vi "Hysteresis.vi"() -> ()   [LabVIEW 2016]
uses:
  controls/HysteresisCtl.ctl
  controls/Enum.ctl
  libgwyscan-1.2-labview2015-win32/controls/parameters for save Gwyddion arrays.ctl
  <vilib>/Analysis/baseanly.llb/Mean (DBL).vi
  <vilib>/Utility/file.llb/Read Delimited Spreadsheet (string).vi
  <vilib>/Utility/error.llb/Error Cluster From Error Code.vi
  <vilib>/rvi/errors/niLvFpgaAdjustHostInterfaceError.vi
  <vilib>/rvi/interface/nirviReadWriteControl/nirviReadWriteControl.xnode
  controls/FPGAVIreferenceTypeDef.ctl
  FPGA Bitfiles/qnmController797_usbRIO_controllerFPGAmu.lvbitx
  <vilib>/Analysis/NI_AALBase.lvlib
  <vilib>/Analysis/NI_AALPro.lvlib
  NiFpgaLv.dll
panel:
  out "bwd":dbl[](array[numeric]) format="%#.4g"
  in  "Processing":u16(ring) items=["None", "Offset", "Line", "Polynom"]
  in  "Frame":bool=TRUE
  in  "rel Range":dbl=1.0 format="%#_13g"
  in  "fwd":path
  in  "bwd":path
  out "Corrected":T1
  out "Raw":cluster{"fwd raw":dbl[][], "bwd raw":dbl[][]}
  in  "Picture Parameters (to save)":T2={"Width"=0.000136, "Height"=0.000136, "Pixels/Line"=0.0, "Lines"=0.0}
  in  "Data source":enum32{"File", "Internal"}(radio)
  in  "Save":bool
  out "fwd":dbl[](array[numeric]) format="%#.4g"
  in  "Update Hysteresis":bool
  in  "Upload":bool
  in  "Hypothesis":T3(ring)=enum."2nd esti"
  in  "Display Correction":bool
  # "Polynom\ncoeff : a+bx\n+cx2+dx3"
  # "up"
  # "down"
  # "Path (txt/dat)"
  # "Corrected"
  # "Raw"
  # "Forward"
  # "Backward"
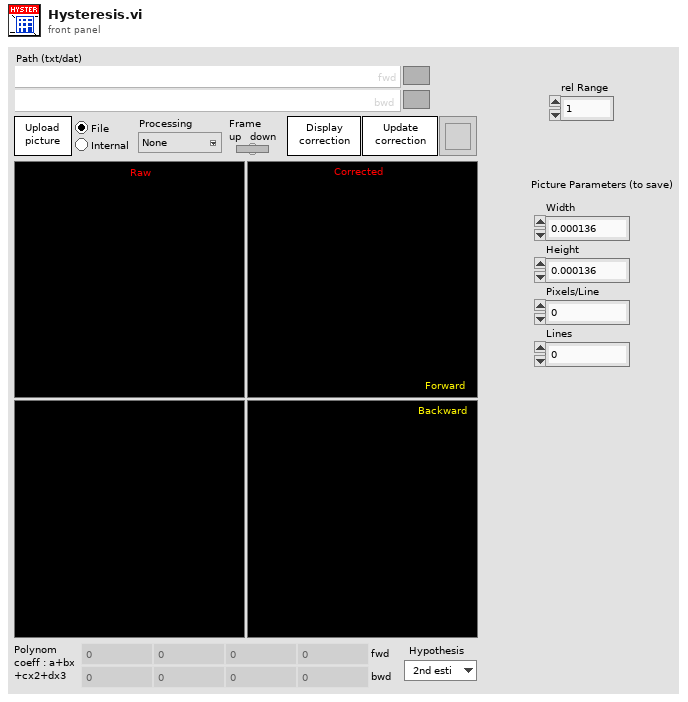
[diagram p1: front panel]
types:
  T1 = cluster{"fwd corrected":dbl[][], "bwd corrected":dbl[][]}
  T2 = cluster{"Width":dbl, "Height":dbl, "Pixels/Line":dbl, "Lines":dbl}
  T3 = enum16{"bwd", "middle", "fwd", "linear", "2nd esti"}
  T4 = typedef "HysteresisCtl.ctl" = enum16{"Init", "Display Correction", "Upload Picture", "Update Hysteresis", "WaitForEvents", "Change.Hypothesis", "Save", "Close"}
  T5 = typedef "Enum.ctl" = enum16{"Init", "Read", "Write"}
  T6 = cluster{"write":bool, "index":u16, "data":fxp<+/-,18,5>}
  T7 = typedef "parameters for save Gwyddion arrays.ctl" = cluster{"X res":i32, "Y res ":i32, "xreal":dbl, "yreal":dbl, "nChannels":i32, "filename":string, "Descriptions":string[], "xyunit":string[], "Z unit":string[]}
  T8 = cluster{"Waveform Shape Fast In":dbl[], "Waveform Shape Slow In":dbl[]}
  T9 = typedef "FPGAVIreferenceTypeDef.ctl" = refnum<k20>
  T10 = cluster{"se.p.enable":bool, "se.p.singleDirection":bool, "se.p.haltScan":bool, "se.mot.p.start":bool}
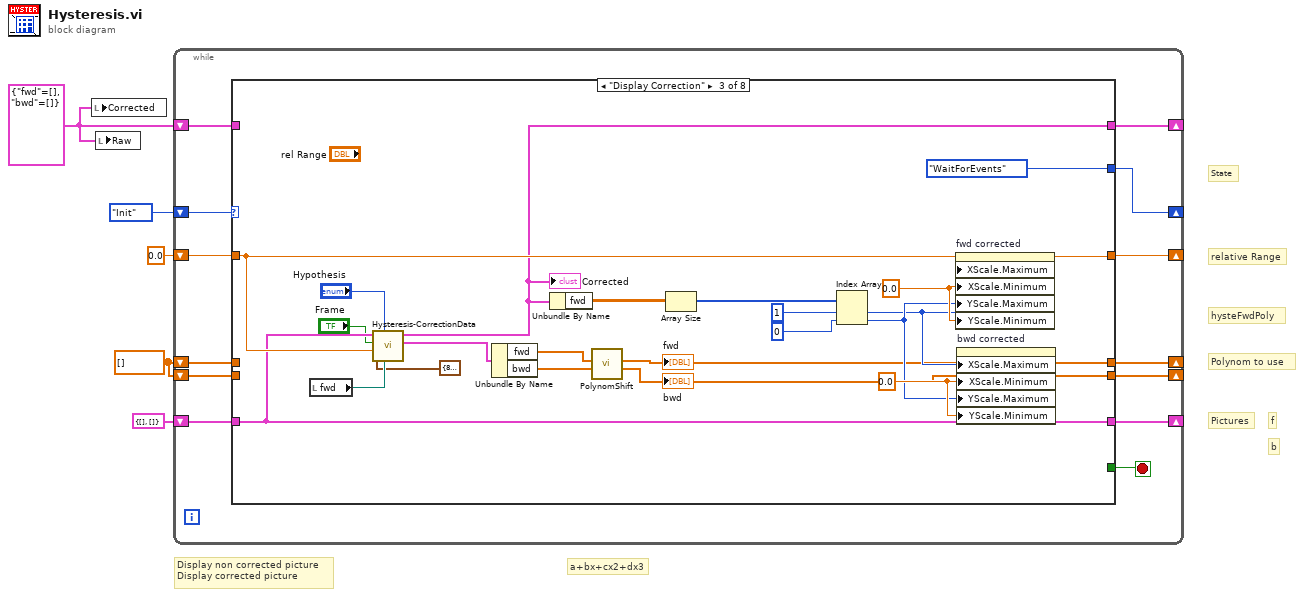
[diagram p0: block diagram]
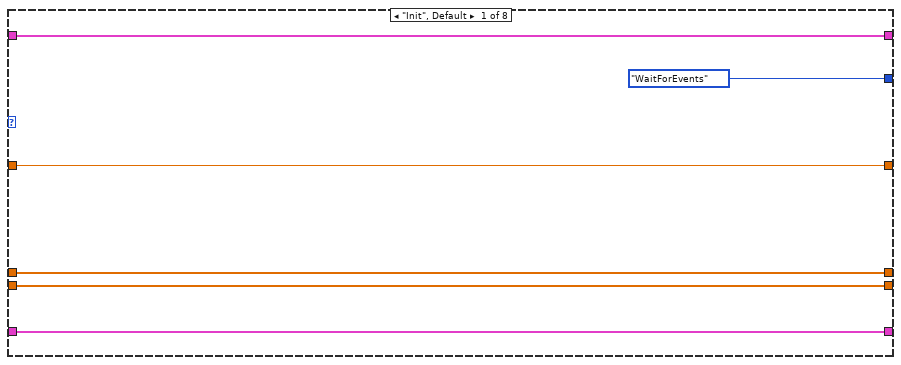
[diagram p2: hidden frame]
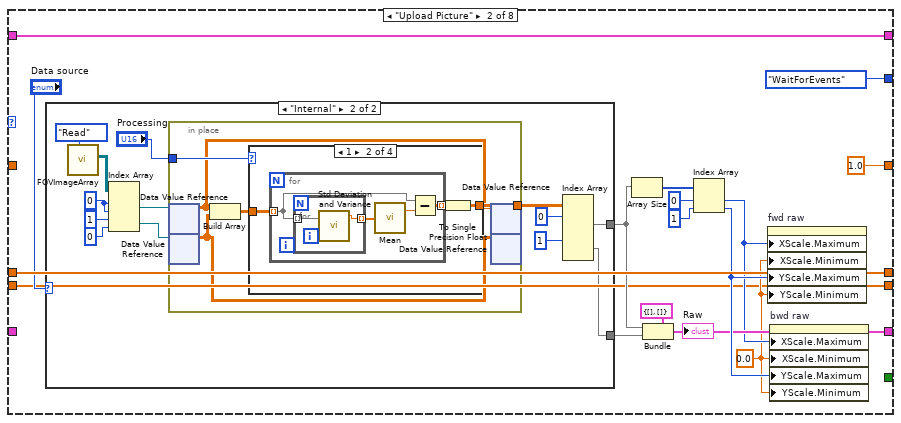
[diagram p3: hidden frame]
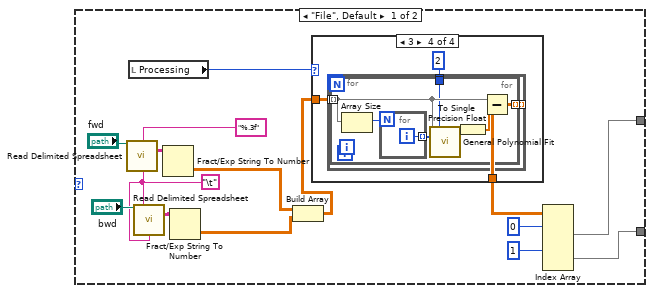
[diagram p4: hidden frame]
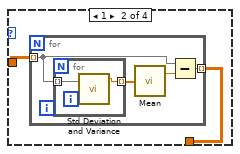
[diagram p6: hidden frame]
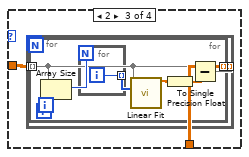
[diagram p7: hidden frame]
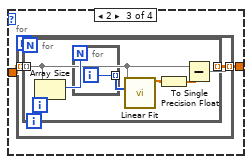
[diagram p9: hidden frame]
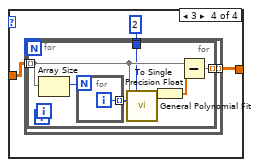
[diagram p10: hidden frame]
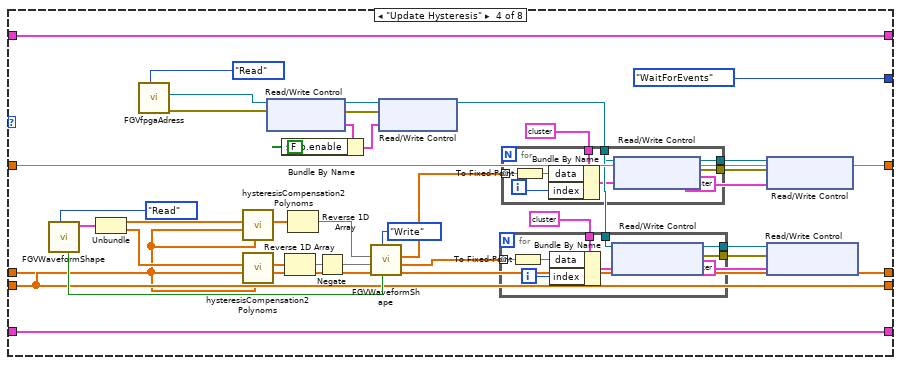
[diagram p11: hidden frame]
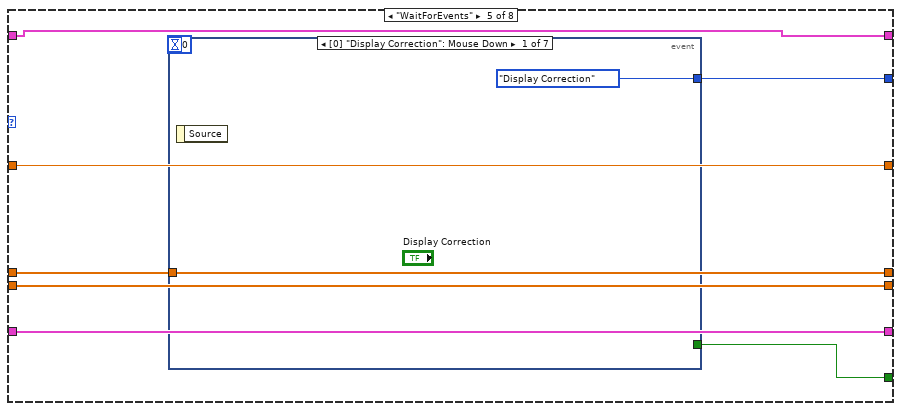
[diagram p12: hidden frame]
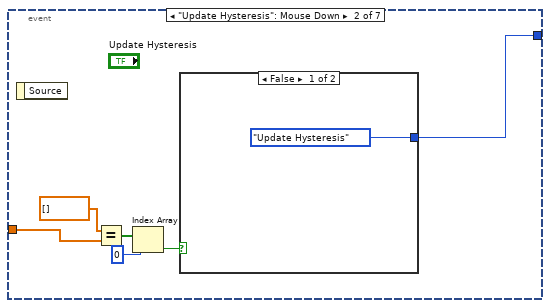
[diagram p13: hidden frame]
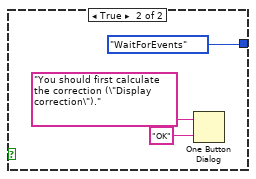
[diagram p14: hidden frame]
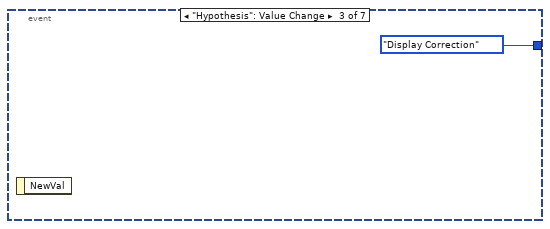
[diagram p15: hidden frame]
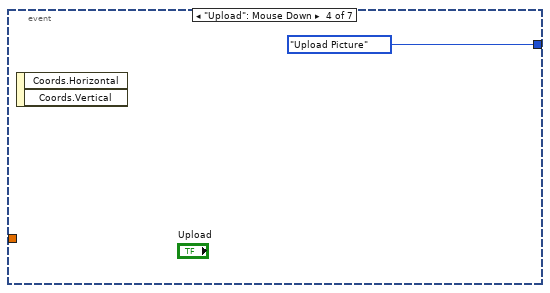
[diagram p16: hidden frame]
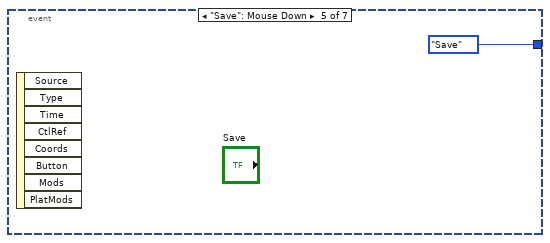
[diagram p17: hidden frame]
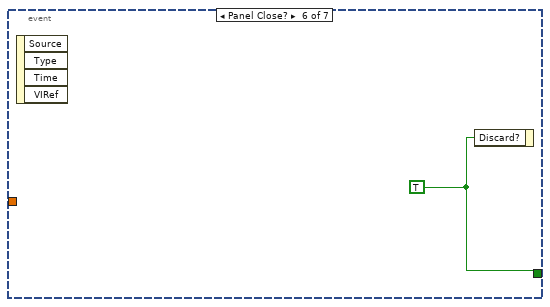
[diagram p18: hidden frame]
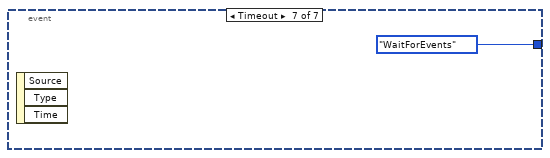
[diagram p19: hidden frame]
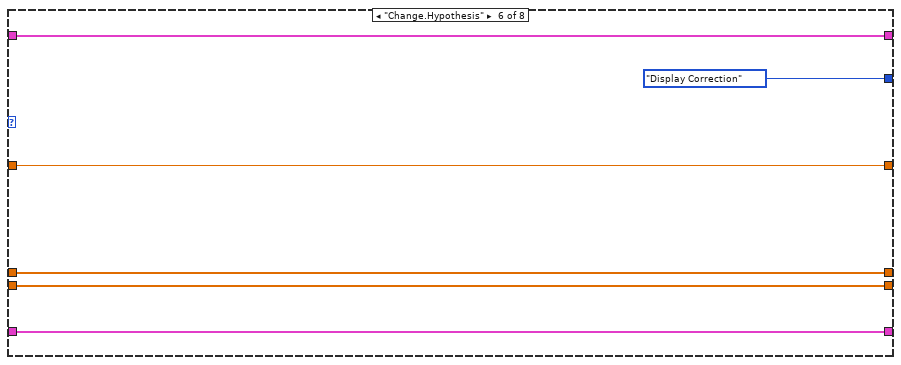
[diagram p20: hidden frame]
diagram:
  w2 = cluster{"fwd":dbl[][], "bwd":dbl[][]} {"fwd"=[], "bwd"=[]} ("cluster")
  w1 = dbl[] [] ("Polynomial Coefficients fwd")
  # "a+bx+cx2+dx3"
  # "Polynom to use"
  # "b"
  # "f"
  # "State"
  # "Pictures"
  # "hysteFwdPoly"
  # "relative Range"
  # "Display non corrected picture\nDisplay corrected picture"
  n1 = local write "Corrected"(w2) -> ()
  n2 = local write "Raw"(w2) -> ()
  n3 = while {
    shift-right: [w16] -> _
    shift-left: HysteresisCtl."Init" -> [w18]
    shift-right: [w15] -> _
    shift-left: cluster{"fwd":dbl[][], "bwd":dbl[][]} {"fwd"=[], "bwd"=[]} ("cluster") -> [w12]
    shift-right: [w14] -> _
    shift-left: 0.0 -> [w13]
    shift-right: [w11] -> _
    shift-left: w1 -> [w10]
    shift-right: [w9] -> _
    shift-left: w2 -> [w8]
    shift-right: [w7] -> _
    shift-left: w1 -> [w6]
    stop <- w17 stop-if-true
    n4 = case shown="\"Display Correction\"" w18 {
      tunnel: [_ _ _ _ w219 _ _ TRUE] -> w17
      tunnel: [HysteresisCtl."WaitForEvents" HysteresisCtl."WaitForEvents" HysteresisCtl."WaitForEvents" HysteresisCtl."WaitForEvents" w221 HysteresisCtl."Display Correction" HysteresisCtl."WaitForEvents" HysteresisCtl."WaitForEvents"] -> w16
      tunnel: [w23 w36 w156 w198 w222 w244 w247 w299] -> w15
      tunnel: [w24 1.0 w163 w199 w223 w245 w282 w300] -> w14
      tunnel: w13 -> [w24 _ w163 w199 w223 w245 w282 w300]
      tunnel: w12 -> [w23 _ w156 w198 w222 w244 w247 w299]
      tunnel: [w19 w40 w145 w177 w220 w243 w281 w298] -> w11
      tunnel: w10 -> [w19 w40 _ w167 w220 w243 w281 w298]
      tunnel: [w21 w27 w152 w190 w217 w241 w248 w296] -> w9
      tunnel: w8 -> [w21 w27 _ w190 w217 w241 w248 w296]
      tunnel: [w20 w25 w146 w177 w216 w240 w246 w295] -> w7
      tunnel: w6 -> [w20 w25 _ w177 w216 w240 w246 w295]
      frame "Init", Default {
      }
      frame "Upload Picture" {
        w26 = 0.0 ("X Scale.Range:Minimum")
        n5 = case shown="\"Internal\"" "Data source" {
          tunnel: [w42 w93] -> w37
          tunnel: [w43 w94] -> w32
          frame "File", Default {
            w50 = "\t"
            n6 = call-poly <vilib>:"Read Delimited Spreadsheet.vi"("file path (dialog if empty)"="fwd", "delimiter (\\t)"=w50) -> ("all rows"=w55:string[][])  [unwired: 8 in, 5 out]
            n7 = local read "Processing"() -> (w46:u16)
            n8 = call-poly <vilib>:"Read Delimited Spreadsheet.vi"("file path (dialog if empty)"="bwd", "format (%s)"="%.3f", "delimiter (\\t)"=w50) -> ("all rows"=w52:string[][])  [unwired: 7 in, 5 out]
            n9 = Fract/Exp String To Number(string=w55) -> (number=w45:dbl[][])  [unwired: 3 in, 1 out]
            n10 = Fract/Exp String To Number(string=w52) -> (number=w44:dbl[][])  [unwired: 3 in, 1 out]
            n11 = Build Array(w45, w44) -> (w41:dbl[][][])
            n12 = case "Processing : Planefit (for FWD & BWD" shown="3" w46 {
              tunnel: [w56 w57 w66 w78] -> w49
              tunnel: w41 -> [w56 w58 w65 w77]
              frame 0, Default {
              }
              frame 1 {
                n13 = for {
                  tunnel: w58 -> [w61] mode=indexing
                  tunnel: [w59] -> w57 mode=indexing
                  n14 = for {
                    tunnel: w61 -> [w63] mode=indexing
                    tunnel: [w64] -> w60 mode=indexing
                    n15 = call <vilib>:"Std Deviation and Variance.vi"("X"=w63) -> ("mean"=w64:dbl)  [unwired: 1 in, 2 out]
                  }
                  n16 = call-poly <vilib>:"Mean.vi"("X"=w60) -> ("mean"=w62:dbl)  [unwired: 1 out]
                  n17 = Subtract(x=w61, y=w62) -> (x-y=w59:dbl[][])
                }
              }
              frame 2 {
                n18 = for {
                  tunnel: w65 -> [w68] mode=indexing
                  tunnel: [w67] -> w66 mode=indexing
                  n19 = for {
                    tunnel: w68 -> [w70] mode=indexing
                    tunnel: [w69] -> w67 mode=indexing
                    n20 = Array Size(array=w70) -> (size(s)=w71:i32)
                    n21 = for {
                      N: w71 -> [_]
                      tunnel: [w75] -> w72 mode=indexing
                      i -> [w75]
                    }
                    n22 = call <vilib>:"Linear Fit.vi"("Y"=w70, "X"=w72) -> ("Best Linear Fit"=w73:dbl[])  [unwired: 9 in, 4 out]
                    n23 = To Single Precision Float(number=w73) -> (single precision float=w74:sgl[])
                    n24 = Subtract(x=w70, y=w74) -> (x-y=w69:dbl[])
                  }
                }
              }
              frame 3 {
                n25 = for {
                  tunnel: [w81] -> w78 mode=indexing
                  tunnel: w77 -> [w80] mode=indexing
                  tunnel: 2 ("polynomial order") -> [w79]
                  n26 = for {
                    tunnel: w80 -> [w84] mode=indexing
                    tunnel: [w83] -> w81 mode=indexing
                    tunnel: w79 -> [w82]
                    n27 = Array Size(array=w84) -> (size(s)=w85:i32)
                    n28 = for {
                      N: w85 -> [_]
                      tunnel: [w89] -> w86 mode=indexing
                      i -> [w89]
                    }
                    n29 = call <vilib>:"General Polynomial Fit.vi"("Y"=w84, "polynomial order"=w82, "X"=w86) -> ("Best Polynomial Fit"=w87:dbl[])  [unwired: 9 in, 3 out]
                    n30 = To Single Precision Float(number=w87) -> (single precision float=w88:sgl[])
                    n31 = Subtract(x=w84, y=w88) -> (x-y=w83:dbl[])
                  }
                }
              }
            }
            n32 = Index Array(array=w49, index (dim 0) #1=0 ("index (page)"), index (dim 0) #2=1 ("index (page)")) -> (element #1=w43:dbl[][], element #2=w42:dbl[][])  [unwired: 4 in]
          }
          frame "Internal" {
            w101 = 0 ("index (vol)")
            n33 = call "FGVImageArray.vi"("Enum"=Enum."Read") -> ("ImageRefOut"=w92:refnum<data-value>[][])  [unwired: 9 in, 1 out]
            n34 = Index Array(array=w92, index (row) #1=w101, index (col) #1=w101, index (row) #2=1 ("index (vol)"), index (col) #2=0 ("disabled index (page)")) -> (element #1=w91:refnum<data-value>, element #2=w90:refnum<data-value>)
            n35 = in-place {
              in-place-border: [w107] -> w96
              in-place-border: "Processing" -> [w106]
              n36 = in-place-dvr #1(w91) -> (w103:sgl[][])  [unwired: 1 out]
              n37 = in-place-dvr #2(w90) -> (w104:sgl[][])  [unwired: 1 out]
              n38 = Build Array(w103, w104) -> (w105:sgl[][][])
              n39 = case "Processing : Planefit (for FWD & BWD" shown="1" w106 {
                tunnel: [w108 w109 w119 w131] -> w107
                tunnel: w105 -> [w108 w111 w118 w130]
                frame 0, Default {
                }
                frame 1 {
                  n40 = for {
                    tunnel: w111 -> [w114] mode=indexing
                    tunnel: [w112] -> w110 mode=indexing
                    n41 = for {
                      tunnel: w114 -> [w116] mode=indexing
                      tunnel: [w117] -> w113 mode=indexing
                      n42 = call <vilib>:"Std Deviation and Variance.vi"("X"=w116) -> ("mean"=w117:dbl)  [unwired: 1 in, 2 out]
                    }
                    n43 = call-poly <vilib>:"Mean.vi"("X"=w113) -> ("mean"=w115:dbl)  [unwired: 1 out]
                    n44 = Subtract(x=w114, y=w115) -> (x-y=w112:dbl[][])
                  }
                  n45 = To Single Precision Float(number=w110) -> (single precision float=w109:sgl[][][])
                }
                frame 2 {
                  n46 = for {
                    tunnel: w118 -> [w121] mode=indexing
                    tunnel: [w120] -> w119 mode=indexing
                    n47 = for {
                      tunnel: w121 -> [w123] mode=indexing
                      tunnel: [w122] -> w120 mode=indexing
                      n48 = Array Size(array=w123) -> (size(s)=w124:i32)
                      n49 = for {
                        N: w124 -> [_]
                        tunnel: [w128] -> w125 mode=indexing
                        i -> [w128]
                      }
                      n50 = call <vilib>:"Linear Fit.vi"("Y"=w123, "X"=w125) -> ("Best Linear Fit"=w126:dbl[])  [unwired: 9 in, 4 out]
                      n51 = To Single Precision Float(number=w126) -> (single precision float=w127:sgl[])
                      n52 = Subtract(x=w123, y=w127) -> (x-y=w122:sgl[])
                    }
                  }
                }
                frame 3 {
                  n53 = for {
                    tunnel: [w134] -> w131 mode=indexing
                    tunnel: w130 -> [w133] mode=indexing
                    tunnel: 2 ("polynomial order") -> [w132]
                    n54 = for {
                      tunnel: w133 -> [w137] mode=indexing
                      tunnel: [w136] -> w134 mode=indexing
                      tunnel: w132 -> [w135]
                      n55 = Array Size(array=w137) -> (size(s)=w138:i32)
                      n56 = for {
                        N: w138 -> [_]
                        tunnel: [w142] -> w139 mode=indexing
                        i -> [w142]
                      }
                      n57 = call <vilib>:"General Polynomial Fit.vi"("Y"=w137, "polynomial order"=w135, "X"=w139) -> ("Best Polynomial Fit"=w140:dbl[])  [unwired: 9 in, 3 out]
                      n58 = To Single Precision Float(number=w140) -> (single precision float=w141:sgl[])
                      n59 = Subtract(x=w137, y=w141) -> (x-y=w136:sgl[])
                    }
                  }
                }
              }
              n60 = in-place-dvr #1(w103) -> ()  [unwired: 2 out]
              n61 = in-place-dvr #2(w104) -> ()  [unwired: 2 out]
            }
            n62 = Index Array(array=w96, index (dim 0) #1=0 ("index (page)"), index (dim 0) #2=1 ("index (page)")) -> (element #1=w94:sgl[][], element #2=w93:sgl[][])  [unwired: 4 in]
          }
        }
        n63 = Array Size(array=w32) -> (size(s)=w31:i32[])
        n64 = Bundle(cluster=cluster{"fwd":dbl[][], "bwd":dbl[][]} {"fwd"=[], "bwd"=[]}, "fwd"=w32, "bwd"=w37) -> (w36:cluster{"fwd":dbl[][], "bwd":dbl[][]})
        "Raw" <- w36
        n65 = Index Array(array=w31, index #1=0 ("index"), index #2=1 ("index")) -> (element #1=w28:i32, element #2=w39:i32)
        n66 = property on="fwd raw" class="IntGraph (strict)"("XScale.Maximum"=w28, "XScale.Minimum"=w26, "YScale.Maximum"=w39, "YScale.Minimum"=w26) -> ()  [unwired: 2 in, 2 out]
        n67 = property on="bwd raw" class="IntGraph (strict)"("XScale.Maximum"=w28, "XScale.Minimum"=w26, "YScale.Maximum"=w39, "YScale.Minimum"=w26) -> ()  [unwired: 2 in, 2 out]
      }
      frame "Display Correction" {
        w160 = 0.0
        w161 = 0.0
        n68 = local read "fwd"() -> (w149:path)
        n69 = call "Hysteresis-CorrectionData.vi"("path"=w149, "hypothesis"="Hypothesis", "Picture Parameters (to save)"=cluster{"Width":dbl, "Height":dbl} {"Width"=8e-05, "Height"=8e-05}, "rel Range"=w163, "Frame"="Frame", "Raw 2"=w156) -> ("Polynomial Coefficients"=w147:cluster{"fwd":dbl[], "bwd":dbl[]}, "Corrected"=w152:cluster{"fwd":dbl[][], "bwd":dbl[][]})  [unwired: 1 in, 3 out]
        "Corrected" <- w152
        n70 = Unbundle By Name(w147) -> ("fwd"=w144:dbl[], "bwd"=w143:dbl[])
        n71 = Unbundle By Name(w152) -> ("fwd"=w155:dbl[][])
        n72 = call "PolynomShift.vi"("CoefficientsBwd"=w143, "CoefficientsFwd"=w144) -> ("ShiftedCoefficientsBwd"=w146:dbl[], "ShiftedCoefficientsFwd"=w145:dbl[])  [unwired: 7 in, 1 out]
        "fwd" <- w145
        "bwd" <- w146
        n73 = Array Size(array=w155) -> (size(s)=w153:i32[])
        n74 = Index Array(array=w153, index #1=1 ("index"), index #2=0 ("index")) -> (element #1=w150:i32, element #2=w151:i32)
        n75 = property on="fwd corrected" class="IntGraph (strict)"("XScale.Maximum"=w150, "XScale.Minimum"=w161, "YScale.Maximum"=w151, "YScale.Minimum"=w161) -> ()  [unwired: 2 in, 2 out]
        n76 = property on="bwd corrected" class="IntGraph (strict)"("XScale.Maximum"=w150, "XScale.Minimum"=w160, "YScale.Maximum"=w151, "YScale.Minimum"=w160) -> ()  [unwired: 2 in, 2 out]
      }
      frame "Update Hysteresis" {
        n77 = call "FGVWaveformShape.vi"("Enum"=Enum."Read") -> ("WaveformInit"=w197:T8, "Framing up? (down: f) out"=w189:bool)  [unwired: 6 in, 3 out]
        n78 = Unbundle(w197) -> ("Waveform Shape Fast In"=w187:dbl[], "Waveform Shape Slow In"=w168:dbl[])
        n79 = call "FGVfpgaAdress.vi"("Enum"=Enum."Read") -> ("error out"=w185:errorcluster, "FPGA VI Reference Out"=w184:T9)  [unwired: 5 in, 4 out]
        n80 = call "hysteresisCompensation2Polynoms.vi"("PolynomBWD"=w167, "PolynomFWD"=w167, "Uncorrected Shape"=w187) -> ("Corrected Shape"=w188:dbl[])  [unwired: 7 in, 1 out]
        n81 = call "hysteresisCompensation2Polynoms.vi"("PolynomBWD"=w167, "PolynomFWD"=w167, "Uncorrected Shape"=w168) -> ("Corrected Shape"=w164:dbl[])  [unwired: 7 in, 1 out]
        n82 = xnode "Read/Write Control"("FPGA VI Reference In"=w184, "error in"=w185) -> ("FPGA VI Reference Out"=w183:T9, "error out"=w182:errorcluster, "se.p.modes"=w181:T10)
        n83 = Bundle By Name(cluster=w181, "se.p.enable"=FALSE ("scanEnabled")) -> (w179:T10)
        n84 = Reverse 1D Array(array=w164) -> (reversed array=w166:dbl[])
        n85 = Reverse 1D Array(array=w188) -> (reversed array=w178:dbl[])
        n86 = Negate(x=w166) -> (-x=w165:dbl[])
        n87 = call "FGVWaveformShape.vi"("Framing up? (down: f) In"=w189, "Enum"=Enum."Write", "Waveform Shape Slow In"=w165, "Waveform Shape Fast In"=w178) -> ("Waveform Shape Slow Out"=w193:dbl[], "Waveform Shape Fast Out"=w194:dbl[])  [unwired: 3 in, 3 out]
        n88 = xnode "Read/Write Control"("FPGA VI Reference In"=w183, "error in"=w182, "se.p.modes"=w179) -> ("FPGA VI Reference Out"=w192:T9)  [unwired: 1 out]
        n89 = for {
          tunnel: [w206] -> w171
          tunnel: w193 -> [w205] mode=indexing
          tunnel: T6 {"write"=TRUE, "index"=0, "data"=0.0} ("slowWaveWrite") -> [w201]
          tunnel: w192 -> [w204]
          tunnel: [w207] -> w172
          i -> [w200]
          n90 = To Fixed-Point(number=w205) -> (fixed-point=w202:fxp<+/-,18,5>)  [unwired: 1 in]
          n91 = Bundle By Name(cluster=w201, "data"=w202, "index"=w200) -> (w203:T6)
          n92 = xnode "Read/Write Control"("FPGA VI Reference In"=w204, "se.m.slowAxis"=w203) -> ("FPGA VI Reference Out"=w207:T9, "error out"=w206:errorcluster)  [unwired: 1 in]
        }
        n93 = for {
          tunnel: [w214] -> w174
          tunnel: w194 -> [w213] mode=indexing
          tunnel: T6 {"write"=TRUE, "index"=0, "data"=0.0} ("slowWaveWrite") -> [w209]
          tunnel: w192 -> [w212]
          tunnel: [w215] -> w175
          i -> [w208]
          n94 = To Fixed-Point(number=w213) -> (fixed-point=w210:fxp<+/-,18,5>)  [unwired: 1 in]
          n95 = Bundle By Name(cluster=w209, "data"=w210, "index"=w208) -> (w211:T6)
          n96 = xnode "Read/Write Control"("FPGA VI Reference In"=w212, "se.m.fastAxis"=w211) -> ("FPGA VI Reference Out"=w215:T9, "error out"=w214:errorcluster)  [unwired: 1 in]
        }
        n97 = xnode "Read/Write Control"("FPGA VI Reference In"=w175, "error in"=w174, "se.m.fastAxis"=T6 {"write"=FALSE, "index"=0, "data"=0.0} ("fastWaveWrite")) -> ()  [unwired: 2 out]
        n98 = xnode "Read/Write Control"("FPGA VI Reference In"=w172, "error in"=w171, "se.m.slowAxis"=T6 {"write"=FALSE, "index"=0, "data"=0.0} ("fastWaveWrite")) -> ()  [unwired: 2 out]
      }
      frame "WaitForEvents" {
        n99 = event shown="[0] \"Display Correction\": Mouse Down" {
          selector: _ -> [_ _ _ _ _ _ _]
          dyn-events: _ -> [_ _ _ _ _ _ _]
          timeout: 200 -> [_ _ _ _ _ _ _]
          tunnel: [HysteresisCtl."Display Correction" w228 HysteresisCtl."Display Correction" HysteresisCtl."Upload Picture" HysteresisCtl."Save" _ HysteresisCtl."WaitForEvents"] -> w221
          tunnel: w220 -> [_ w229 _ _ _ _ _]
          tunnel: [_ _ _ _ _ w238 _] -> w219
          event "Display Correction": Mouse Down {
            n100 = event-data() -> ()  [unwired: 1 in, 1 out]
          }
          event "Update Hysteresis": Mouse Down {
            n101 = event-data() -> ()  [unwired: 1 in, 1 out]
            n102 = Equal?(x=dbl[] [] ("Polynomial Coefficients fwd"), y=w229) -> (x = y?=w226:bool[])
            n103 = Index Array(array=w226, index=0) -> (element=w227:bool)
            n104 = case shown="False" w227 {
              tunnel: [HysteresisCtl."Update Hysteresis" HysteresisCtl."WaitForEvents"] -> w228
              frame False {
              }
              frame True {
                n105 = One Button Dialog(message="You should first calculate the correction (\"Display correction\").", button name ("OK")="OK") -> ()  [unwired: 1 out]
              }
            }
          }
          event "Hypothesis": Value Change {
            n106 = event-data() -> ()  [unwired: 1 in, 1 out]
          }
          event "Upload": Mouse Down {
            n107 = event-data() -> ()  [unwired: 1 in, 2 out]
          }
          event "Save": Mouse Down {
            n108 = event-data() -> ()  [unwired: 1 in, 8 out]
          }
          event Panel Close? {
            w238 = TRUE
            n109 = event-data() -> ()  [unwired: 1 in, 4 out]
            n110 = event-data("Discard?"=w238) -> ()  [unwired: 1 in, 1 out]
          }
          event Timeout {
            n111 = event-data() -> ()  [unwired: 1 in, 3 out]
          }
        }
      }
      frame "Change.Hypothesis" {
      }
      frame "Save" {
        # "Save the picture"
        n112 = Unbundle(w247) -> ("fwd"=w249:dbl[][], "bwd"=w252:dbl[][])
        n113 = Array Size(array=w249) -> (size(s)=w251:i32[])
        n114 = Build Array(w249, w252) -> (w268:dbl[][][])
        n115 = local read "fwd"() -> (w250:path)
        n116 = for {
          N: 2 -> [_]
          tunnel: w268 -> [w294]
          tunnel: [w291] -> w273 mode=concatenating
          tunnel: [w288] -> w274 mode=indexing
          tunnel: ["m"] -> w275 mode=indexing
          tunnel: [w284] -> w276 mode=indexing
          tunnel: "m" -> [w284]
          i -> [w289]
          n117 = Equal To 0?(x=w289) -> (x = 0?=w290:bool)
          n118 = Index Array(array=w294, index (dim 0)=w289) -> (element=w292:dbl[][])  [unwired: 2 in]
          n119 = Array Size(array=w292) -> (size(s)=w287:i32[])
          n120 = Multiply Array Elements(1:w287) -> (0:w293:i32)
          n121 = Select(t="[Fwd]", s=w290, f="[Bwd]") -> (s? t:f=w288:string)
          n122 = Reshape Array(w292, w293) -> (w291:dbl[])
        }
        n123 = Strip Path(path=w250) -> (stripped path=w261:path, name=w255:string)
        n124 = Match Pattern(string=w255, regular expression=".txt") -> (before substring=w253:string)  [unwired: 1 in, 3 out]
        n125 = Concatenate Strings(w253, "corrected.gwy" ("filename")) -> (w263:string)
        n126 = Build Path(base path=w261, name or relative path=w263) -> (appended path=w265:path)
        n127 = Index Array(array=w251, index #1=0 ("index"), index #2=1 ("index")) -> (element #1=w257:i32, element #2=w256:i32)
        n128 = Format Into String(w265) -> (resulting string=w264:string)  [unwired: 3 in, 1 out]
        n129 = Unbundle By Name("Picture Parameters (to save)") -> ("Width"=w277:dbl, "Height"=w278:dbl)
        n130 = To Long Integer(number=w257) -> (32bit integer=w272:i32)
        n131 = To Long Integer(number=w256) -> (32bit integer=w271:i32)
        n132 = Bundle By Name(cluster=T7 {"X res"=0, "Y res "=0, "xreal"=0.0, "yreal"=0.0, "nChannels"=0, "filename"="", "Descriptions"=[], "xyunit"=[], "Z unit"=[]} ("parameters for save Gwyddion arrays"), "xreal"=w277, "yreal"=w278, "X res"=w272, "Y res"=w271, "Descriptions"=w274, "xyunit"=w275, "Z unit"=w276, "nChannels"=2 ("y"), "filename"=w264) -> (w269:T7)
        n133 = call "Access to save gwyddion arrays.vi"("parameters for save Gwyddion arrays"=w269, "data IN"=w273) -> ()  [unwired: 3 in, 1 out]
      }
      frame "Close" {
      }
    }
  }
